vi "OpenMUXChannel.vi"(8 "error in (no error)":errorcluster, 10 "gRPCid":T2, 11 "ctet_mux in":T1) -> (0 "error out":errorcluster, 3 "ctet_mux out":T1)   [LabVIEW 2019, in "ctet_mux_User Library.lvlib"]
uses:
  ctet_mux_User Library.lvlib
  Servers/ctet_mux/gRPC lvSupport/Server API/typeDefs/grpcId.ctl
  Types/ctet_mux.ctl
  Servers/ctet_mux/ctet_mux Class/RPC Messages/measurementservice_MUXOpenChannelResponse/measurementservice_MUXOpenChannelResponse_Data.ctl
  Servers/ctet_mux/ctet_mux Class/RPC Messages/measurementservice_ErrorOut/measurementservice_ErrorOut_Data.ctl
  Types/Switch Action.ctl
  <instrlib>/niSwitch/niSwitch.llb/niSwitch Disconnect Channels (Single).vi
  Servers/ctet_mux/ctet_mux Class/ctet_mux.lvclass
  Servers/ctet_mux/gRPC lvSupport/gprc-lvsupport.lvlib
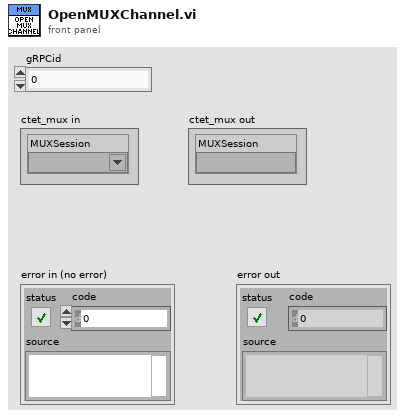
[diagram p1: front panel]
types:
  T1 = typedef "ctet_mux_User Library.lvlib/ctet_mux.ctl" = cluster{"MUXSession":refnum<k15>}
  T2 = typedef "ctet_mux.lvlib/gprc-lvsupport.lvlib/grpcId.ctl" = u64
  T3 = typedef "ctet_mux_User Library.lvlib/Switch Action.ctl" = enum16{"Get Switch State", "Initialize", "Connect Channel", "Open Channel", "Close Relay", "Open Relay", "Disconnect/Open All"}
  T4 = typedef "ctet_mux.lvlib/ctet_mux.lvclass/measurementservice_ErrorOut_Data.ctl" = cluster{"errCode":i64, "errMessage":string}
  T5 = typedef "ctet_mux.lvlib/ctet_mux.lvclass/measurementservice_MUXOpenChannelResponse_Data.ctl" = cluster{"error":T4}
  T6 = typedef "ctet_mux.lvlib/ctet_mux.lvclass/measurementservice_MUXOpenChannelRequest_Data.ctl" = cluster{"Channel1":string, "Channel2":string}
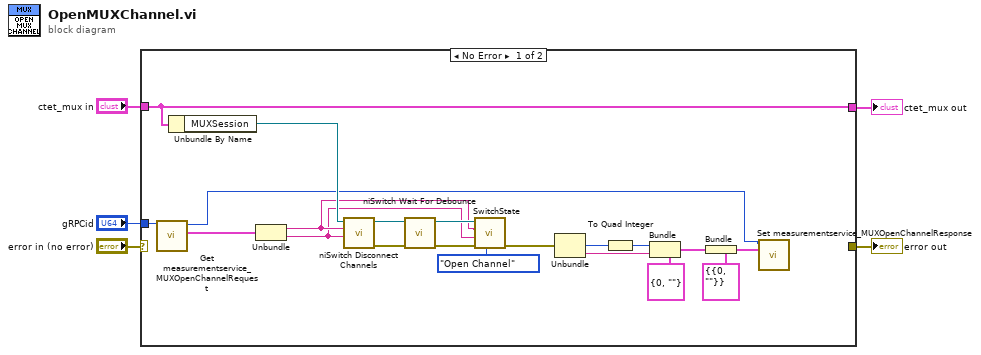
[diagram p0: block diagram]
diagram:
  n1 = case shown="No Error" "error in (no error)" {
    selector: "error in (no error)" -> [_ w27]
    tunnel: [_ w27] -> w5
    tunnel: "gRPCid" -> [w18 _]
    tunnel: "ctet_mux in" -> [w22 w26]
    tunnel: [w22 w26] -> w1
    frame No Error {
      n2 = call "Get measurementservice_MUXOpenChannelRequest.vi"("gRPCid"=w18) -> ("Message Data"=w17:T6, "gRPCid out"=w16:T2)  [unwired: 8 in, 1 out]
      n3 = Unbundle By Name(w22) -> ("MUXSession"=w19:refnum<k15>)
      n4 = Unbundle(w17) -> ("Channel1"=w8:string, "Channel2"=w7:string)
      n5 = call-poly <instrlib>:"niSwitch Disconnect Channels.vi"("channel 2"=w7, "channel 1"=w8, "instrument handle"=w19) -> ("error out"=w20:errorcluster, "instrument handle out"=w21:refnum<k15>)  [unwired: 7 in]
      n6 = call <instrlib>:"niSwitch Wait For Debounce.vi"("error in (no error)"=w20, "instrument handle"=w21) -> ("error out"=w11:errorcluster, "instrument handle out"=w9:refnum<k15>)  [unwired: 8 in]
      n7 = call "SwitchState.vi"("Switch Action"=Switch_Action."Open Channel", "error in (no error)"=w11, "channel 2"=w7, "channel 1"=w8, "Switch Session"=w9) -> ("error out"=w10:errorcluster)  [unwired: 4 in, 2 out]
      n8 = Unbundle(w10) -> ("code"=w24:i32, "source"=w25:string)  [unwired: 1 out]
      n9 = To Quad Integer(1:w24) -> (0:w23:i64)
      n10 = Bundle(cluster=T4 {"errCode"=0, "errMessage"=""} ("error"), "errCode"=w23, "errMessage"=w25) -> (w12:T4)
      n11 = Bundle(cluster=T5 {"error"={"errCode"=0, "errMessage"=""}} ("Message Data"), "error"=w12) -> (w14:T5)
      n12 = call "Set measurementservice_MUXOpenChannelResponse.vi"("Message Data"=w14, "gRPCid"=w16) -> ()  [unwired: 9 in, 1 out]
    }
    frame Error {
    }
  }
  "error out" <- w5
  "ctet_mux out" <- w1
